vi "Translate GPS Data.vi"(0 "Read Buffer":string) -> (20 "Sample Time":string, 21 "Latitude":dbl format="%_13g", 22 "North or South":string, 23 "Longitude":dbl format="%_13g", 24 "East or West":string, 25 "Fixed Quality":string, 26 "Satellites Tracked":string, 27 "Altitude Above Mean Sea Level (m)":string)   [LabVIEW 2011]
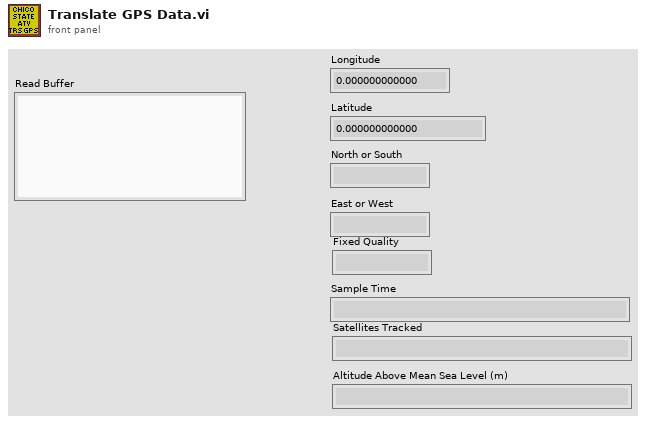
[diagram p1: front panel]
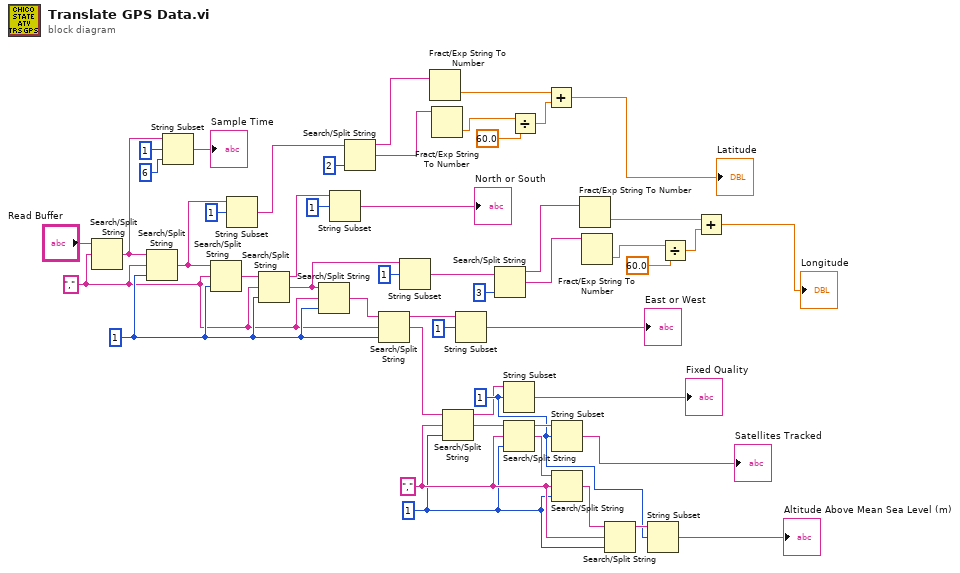
[diagram p0: block diagram]
diagram:
  w27 = 1 ("offset (0)")
  w31 = "," ("search string/char (-)")
  w33 = 1 ("offset (0)")
  w49 = 1 ("offset (0)")
  w34 = "," ("search string/char (-)")
  n1 = Search/Split String(string="Read Buffer", search string/char (-)=w34) -> (match + rest of string=w42:string)  [unwired: 1 in, 2 out]
  n2 = Search/Split String(string=w42, search string/char (-)=w34, offset (0)=w49) -> (match + rest of string=w3:string)  [unwired: 2 out]
  n3 = String Subset(string=w42, offset (0)=1, length (rest)=6 ("length (rest)")) -> (substring=→"Sample Time":string)
  n4 = Search/Split String(string=w3, search string/char (-)=w34, offset (0)=w49) -> (match + rest of string=w50:string)  [unwired: 2 out]
  n5 = String Subset(string=w3, offset (0)=1) -> (substring=w6:string)  [unwired: 1 in]
  n6 = Search/Split String(string=w50, search string/char (-)=w34, offset (0)=w49) -> (substring before match=w47:string, match + rest of string=w1:string)  [unwired: 1 out]
  n7 = Search/Split String(string=w1, search string/char (-)=w34, offset (0)=w49) -> (match + rest of string=w2:string)  [unwired: 2 out]
  n8 = String Subset(string=w47, offset (0)=1 ("length (rest)")) -> (substring=→"North or South":string)  [unwired: 1 in]
  n9 = Search/Split String(string=w6, offset (0)=2) -> (substring before match=w22:string, match + rest of string=w21:string)  [unwired: 1 in, 1 out]
  n10 = Search/Split String(string=w2, search string/char (-)=w34, offset (0)=w49) -> (substring before match=w48:string, match + rest of string=w28:string)  [unwired: 1 out]
  n11 = String Subset(string=w1, offset (0)=1) -> (substring=w5:string)  [unwired: 1 in]
  n12 = Fract/Exp String To Number(string=w22) -> (number=w18:dbl)  [unwired: 3 in, 1 out]
  n13 = Fract/Exp String To Number(string=w21) -> (number=w19:dbl)  [unwired: 3 in, 1 out]
  n14 = Search/Split String(string=w28, search string/char (-)=w31, offset (0)=w27) -> (substring before match=w30:string, match + rest of string=w29:string)  [unwired: 1 out]
  n15 = String Subset(string=w48, offset (0)=1 ("length (rest)")) -> (substring=→"East or West":string)  [unwired: 1 in]
  n16 = Search/Split String(string=w5, offset (0)=3) -> (substring before match=w14:string, match + rest of string=w13:string)  [unwired: 1 in, 1 out]
  n17 = String Subset(string=w30, offset (0)=w33) -> (substring=→"Fixed Quality":string)  [unwired: 1 in]
  n18 = Search/Split String(string=w29, search string/char (-)=w31, offset (0)=w27) -> (substring before match=w40:string, match + rest of string=w39:string)  [unwired: 1 out]
  n19 = Divide(x=w19, y=60.0) -> (x/y=w17:dbl)
  n20 = Add(x=w18, y=w17) -> (x+y=→"Latitude":dbl)
  n21 = String Subset(string=w40, offset (0)=w33) -> (substring=→"Satellites Tracked":string)  [unwired: 1 in]
  n22 = Search/Split String(string=w39, search string/char (-)=w31, offset (0)=w27) -> (match + rest of string=w37:string)  [unwired: 2 out]
  n23 = Fract/Exp String To Number(string=w14) -> (number=w10:dbl)  [unwired: 3 in, 1 out]
  n24 = Fract/Exp String To Number(string=w13) -> (number=w11:dbl)  [unwired: 3 in, 1 out]
  n25 = Search/Split String(string=w37, search string/char (-)=w31, offset (0)=w27) -> (substring before match=w36:string)  [unwired: 2 out]
  n26 = String Subset(string=w36, offset (0)=w33) -> (substring=→"Altitude Above Mean Sea Level (m)":string)  [unwired: 1 in]
  n27 = Divide(x=w11, y=60.0) -> (x/y=w9:dbl)
  n28 = Add(x=w10, y=w9) -> (x+y=→"Longitude":dbl)
